vi "GF_DatapathFromFile.vi"(0 "Config File Path":path=path "C:/Users/basic/Documents/Configuration") -> (1 "DataPath From File":path, 2 "Datapath Success":bool, 3 "error out":errorcluster)   [LabVIEW 2016]
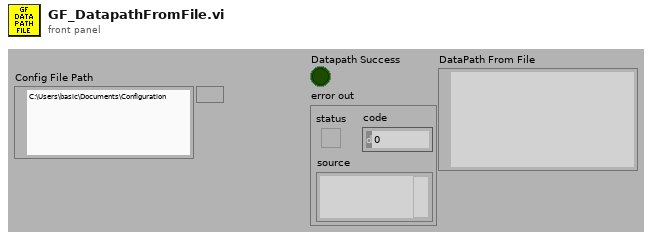
[diagram p1: front panel]
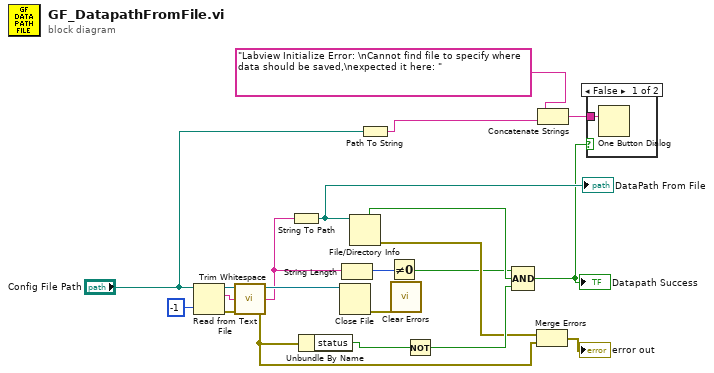
[diagram p0: block diagram]
diagram:
  n1 = Read from Text File(file (use dialog)="Config File Path", count=-1) -> (refnum out=w18:refnum<file>, text=w2:string, error out=w11:errorcluster)  [unwired: 2 in, 1 out]
  n2 = call <vilib>:"Trim Whitespace.vi"("string"=w2) -> ("trimmed string"=w1:string)  [unwired: 1 in]
  n3 = String To Path(string=w1) -> (path=w16:path)
  "DataPath From File" <- w16
  n4 = Unbundle By Name(w11) -> ("status"=w14:bool)
  n5 = Close File(refnum=w18) -> (error out=w17:errorcluster)  [unwired: 1 in, 1 out]
  n6 = String Length(string=w1) -> (length=w4:i32)
  n7 = File/Directory Info(path=w16) -> (directory=w15:bool, error out=w12:errorcluster)  [unwired: 1 in, 5 out]
  n8 = Path To String(path="Config File Path") -> (string=w8:string)
  n9 = Not Equal To 0?(x=w4) -> (x != 0?=w3:bool)
  n10 = call <vilib>:"Clear Errors.vi"("error in (no error)"=w17) -> ()  [unwired: 5 in, 2 out]
  n11 = Not(x=w14) -> (.not. x?=w13:bool)
  n12 = Compound Arithmetic op=AND(w3, w15, w13) -> (w5:bool)
  "Datapath Success" <- w5
  n13 = Merge Errors(w12, w11) -> (→"error out":errorcluster)
  n14 = Concatenate Strings("Labview Initialize Error: \nCannot find file to specify where data should be saved,\nexpected it here: " ("error source (\" \")"), w8) -> (w6:string)
  n15 = case shown="False" w5 {
    tunnel: w6 -> [w20 _]
    frame False {
      n16 = One Button Dialog(message=w20) -> ()  [unwired: 1 in, 1 out]
    }
    frame True {
    }
  }
